vi "init mappings.vi"(8 "error in (no error)":errorcluster, 9 "data allocations":T1, 10 "Scaling configuration":refnum<class "Scaling configuration.lvclass">, 11 "Scaling runtime in":refnum<class "Scaling runtime.lvclass">) -> (0 "error out":errorcluster, 3 "Scaling runtime out":refnum<class "Scaling runtime.lvclass">)   [LabVIEW 2013, in "Scaling runtime.lvclass"]
uses:
  Scaling runtime.lvclass
  configuration/Scaling configuration.lvclass
  <vilib>/NI/Tag Bus Module Framework/channel/data tables.ctl
  <vilib>/NI/Tag Bus/dictionary/data dictionary.lvclass
  <vilib>/NI/Tag Bus/dictionary table pair.ctl
  <vilib>/NI/Tag Bus/table/data table.ctl
  Scaling runtime.lvclass/Scaling runtime.ctl
  <vilib>/NI/Tag Bus/tag/Data Type.ctl
  <vilib>/NI/Tag Bus/tag/tag descriptor.lvclass/tag descriptor.ctl
  <vilib>/NI/Tag Bus/tag/read tag name.vi
  <vilib>/NI/Tag Bus/dictionary/locate tag.vi
  <vilib>/NI/Tag Bus/tag/tag descriptor.lvclass
  <vilib>/NI/Tag Bus/table/data table.lvlib
  <vilib>/NI/Tag Bus/tag bus.lvlib
  <vilib>/NI/Tag Bus Module Framework/channel/TBM channel.lvclass
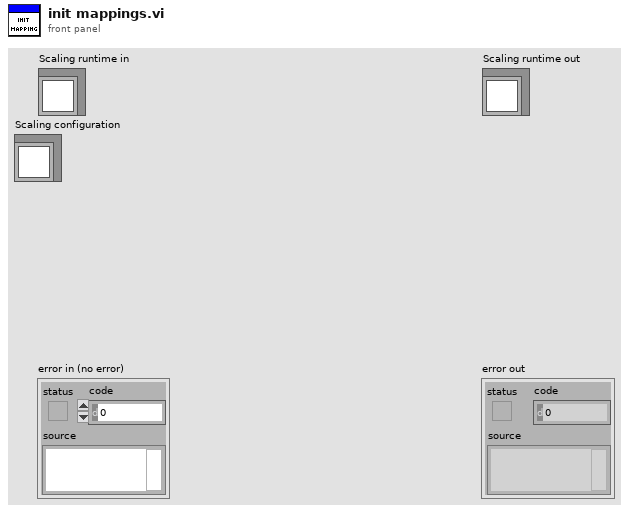
[diagram p1: front panel]
types:
  T1 = typedef "TBM channel.lvclass/data tables.ctl" = cluster{"input data":T2, "processing parameter":T2, "processing result":T2, "output data":T2}
  T2 = typedef "tag bus.lvlib/dictionary table pair.ctl" = cluster{"data dictionary":refnum<class "data dictionary.lvclass">, "data table":T3}
  T3 = typedef "tag bus.lvlib/data table.lvlib/data table.ctl" = cluster{"Double":dbl[], "Single":sgl[], "I64":i64[], "I32":i32[], "I16":i16[], "I8":i8[], "U64":u64[], "U32":u32[], "U16":u16[], "U8":u8[], "Boolean":bool[], "String":string[], "Array of Double":cluster{"DBL Array":dbl[]}[], "Array of Single":cluster{"SGL Array":sgl[]}[], "Array of I64":cluster{"I64 Array":i64[]}[], "Array of I32":cluster{"I32 Array":i32[]}[], "Array of I16":cluster{"I16 Array":i16[]}[], "Array of I8":cluster{"I8 Array":i8[]}[], "Array of U64":cluster{"U64 Array":u64[]}[], "Array of U32":cluster{"U32 Array":u32[]}[], "Array of U16":cluster{"U16 Array":u16[]}[], "Array of U8":cluster{"U8 Array":u8[]}[], "Array of Boolean":cluster{"Boolean Array":bool[]}[], "Array of String":cluster{"String Array":string[]}[]}
  T4 = typedef "tag bus.lvlib/tag descriptor.lvclass/Data Type.ctl" = enum16{"Double", "Single", "I64", "I32", "I16", "I8", "U64", "U32", "U16", "U8", "Boolean", "String", "Array of Double", "Array of Single", "Array of I64", "Array of I32", "Array of I16", "Array of I8", "Array of U64", "Array of U32", "Array of U16", "Array of U8", "Array of Boolean", "Array of String"}
  T5 = cluster{"input channel":refnum<class "TBM channel.lvclass">, "output channel":refnum<class "TBM channel.lvclass">}[][]
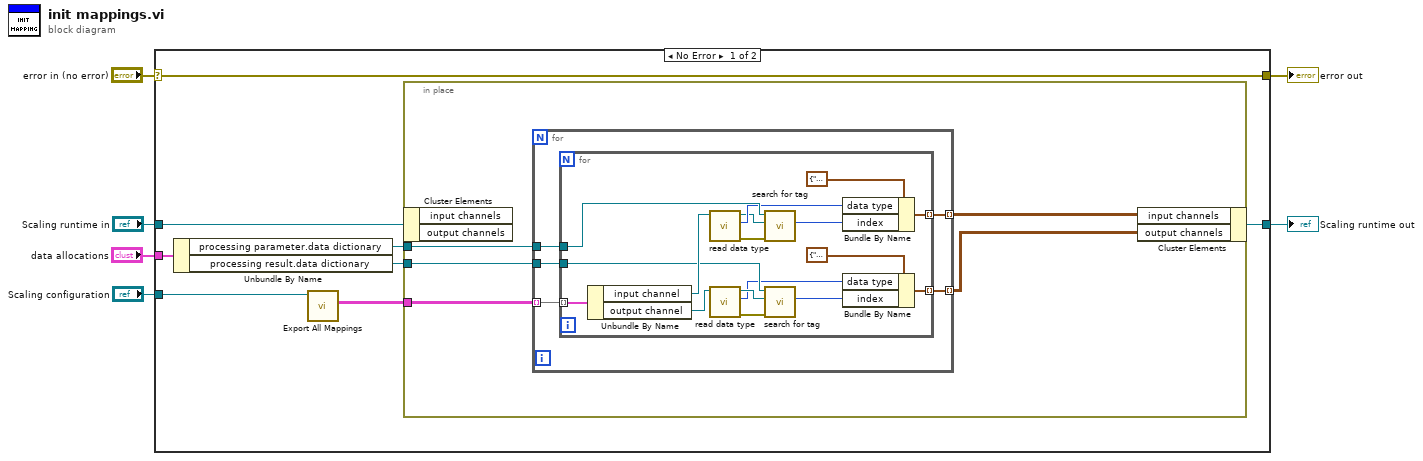
[diagram p0: block diagram]
diagram:
  n1 = case shown="No Error" "error in (no error)" {
    selector: "error in (no error)" -> [w14 w43]
    tunnel: [w14 w43] -> w5
    tunnel: [w7 w42] -> w3
    tunnel: "Scaling runtime in" -> [w11 w42]
    tunnel: "Scaling configuration" -> [w13 _]
    tunnel: "data allocations" -> [w10 _]
    frame No Error {
      n2 = Unbundle By Name(w10) -> ("processing parameter.data dictionary"=w9:refnum<class "data dictionary.lvclass">, "processing result.data dictionary"=w8:refnum<class "data dictionary.lvclass">)
      n3 = call "Export All Mappings.vi"("Scaling configuration in"=w13) -> ("mapping sets"=w12:T5)  [unwired: 8 in, 2 out]
      n4 = in-place {
        in-place-border: w12 -> [w19]
        in-place-border: w9 -> [w18]
        in-place-border: w8 -> [w17]
        n5 = in-place-cluster #1(w11) -> ()  [unwired: 2 out]
        n6 = for {
          tunnel: w19 -> [w24] mode=indexing
          tunnel: w18 -> [w23]
          tunnel: w17 -> [w22]
          tunnel: [w21] -> w16 mode=indexing
          tunnel: [w20] -> w15 mode=indexing
          n7 = for {
            tunnel: w24 -> [w41] mode=indexing
            tunnel: w23 -> [w40]
            tunnel: w22 -> [w32]
            tunnel: [w26] -> w20 mode=indexing
            tunnel: [w25] -> w21 mode=indexing
            n8 = Unbundle By Name(w41) -> ("input channel"=w38:refnum<class "TBM channel.lvclass">, "output channel"=w30:refnum<class "TBM channel.lvclass">)
            n9 = call <vilib>:"read data type.vi"("system tag in"=w38) -> ("error out"=w35:errorcluster, "data type"=w37:T4, "system tag out"=w36:refnum<class "TBM channel.lvclass">)  [unwired: 8 in]
            n10 = call <vilib>:"read data type.vi"("system tag in"=w30) -> ("error out"=w33:errorcluster, "data type"=w27:T4, "system tag out"=w31:refnum<class "TBM channel.lvclass">)  [unwired: 8 in]
            n11 = call <vilib>:"search for tag.vi"("error in"=w35, "system tag"=w36, "data dictionary in"=w40) -> ("index"=w34:i32)  [unwired: 6 in, 2 out]
            n12 = call <vilib>:"search for tag.vi"("error in"=w33, "system tag"=w31, "data dictionary in"=w32) -> ("index"=w28:i32)  [unwired: 6 in, 2 out]
            n13 = Bundle By Name(cluster=cluster{"data type":T4, "index":i32} {"data type"=enum."Double", "index"=0} ("channel"), "data type"=w37, "index"=w34) -> (w25:cluster{"data type":T4, "index":i32})
            n14 = Bundle By Name(cluster=cluster{"data type":T4, "index":i32} {"data type"=enum."Double", "index"=0} ("channel"), "data type"=w27, "index"=w28) -> (w26:cluster{"data type":T4, "index":i32})
          }
        }
        n15 = in-place-cluster #1("input channels"=w16, "output channels"=w15) -> (w7:refnum<class "Scaling runtime.lvclass">)
      }
    }
    frame Error {
    }
  }
  "error out" <- w5
  "Scaling runtime out" <- w3
